vi "Elevator Get Telemetry.vi"() -> (3 "Telemetry":T1)   [LabVIEW 2018]
uses:
  Implementation/Elevator Telemetry.ctl
  Implementation/Elevator Published Globals.vi
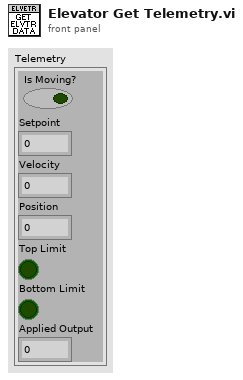
[diagram p1: front panel]
types:
  T1 = typedef "Elevator Telemetry.ctl" = cluster{"Is Moving?":bool, "Setpoint":dbl, "Velocity":dbl, "Position":dbl, "Top Limit":bool, "Bottom Limit":bool, "Applied Output":dbl}
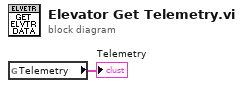
[diagram p0: block diagram]
diagram:
  n1 = global read "Elevator Published Globals.vi" "Telemetry"() -> (→"Telemetry":T1)
